vi "HEWH Temperature Decrease FHD.vi"(7 "error in (no error)":errorcluster) -> (0 "error out":errorcluster, 3 "Temperature Decrease Output":T1 format="%.2f")   [LabVIEW 2019]
uses:
  Utility/Custom Pallet Controls/Custom Pallet DBL.ctl
  Utility/Custom Pallet Controls/Custom Pallet Forward.ctl
panel:
  in  "Tab Control":enum32{"Page 1", "Page 2"}(tab)
  in  "Complete":T2
  in  "Temperature Decrease":T1=15.0 format="%.2f"
  out "Description 2":string="New Standard - 125 Degree Setpoint @ 15 Degree Temperature Decrease\nOld Standard - 135 Degree Setpoint @ 25 Degree Temperature Decrease"
  out "Description":string="Temperature Decrease"
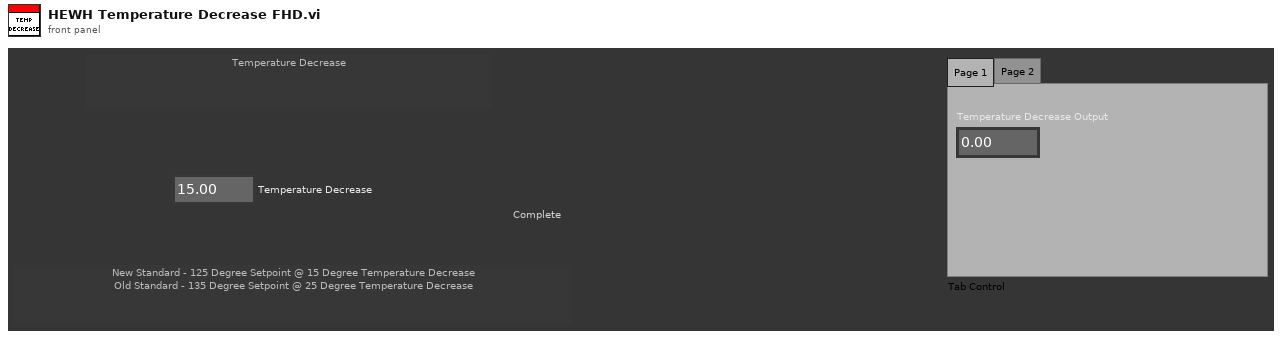
[diagram p1: front panel]
types:
  T1 = typedef "Custom Pallet DBL.ctl" = dbl
  T2 = typedef "Custom Pallet Forward.ctl" = bool
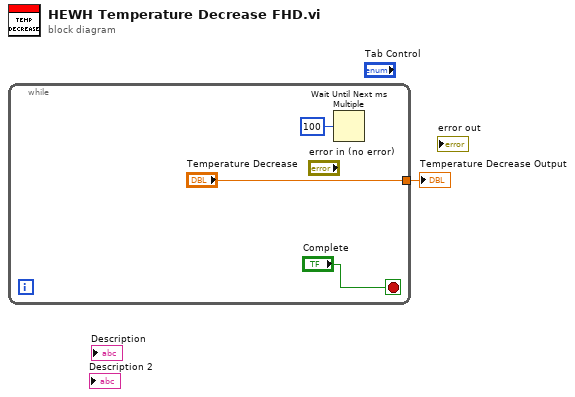
[diagram p0: block diagram]
diagram:
  n1 = while {
    tunnel: ["Temperature Decrease"] -> w1
    stop <- "Complete" stop-if-true
    n2 = Wait Until Next ms Multiple(millisecond multiple=u32 100) -> ()  [unwired: 1 out]
  }
  "Temperature Decrease Output" <- w1
